vi "N04_Math_and_debug.vi"() -> ()   [LabVIEW 2023]
panel:
  out "Multiply":dbl
  out "Subtract":dbl
  out "Add":dbl
  in  "Numeric 2":dbl
  in  "Numeric":dbl
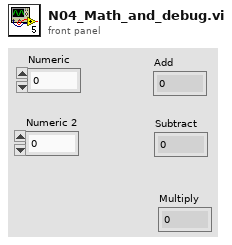
[diagram p1: front panel]
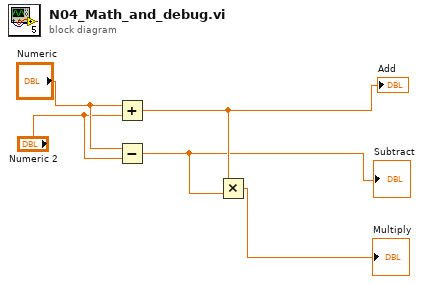
[diagram p0: block diagram]
diagram:
  n1 = Add(x="Numeric", y="Numeric 2") -> (x+y=w2:dbl)
  "Add" <- w2
  n2 = Subtract(x="Numeric", y="Numeric 2") -> (x-y=w1:dbl)
  "Subtract" <- w1
  n3 = Multiply(x=w2, y=w1) -> (x*y=→"Multiply":dbl)
